vi "Scheduler.Clear-Reset.vi"(7 "All Modules(T)/LocalQ(F)":bool, 8 "error in":errorcluster, 11 "Q In":refnum<queue>) -> (0 "error out":errorcluster, 3 "Q Out":refnum<queue>)   [LabVIEW 2024, in "EQMF.lvlib" / "Scheduler.lvlib"]
uses:
  Scheduler.lvlib
  Queues/Q.Element.ctl
  Queues/Queue Utils.lvlib
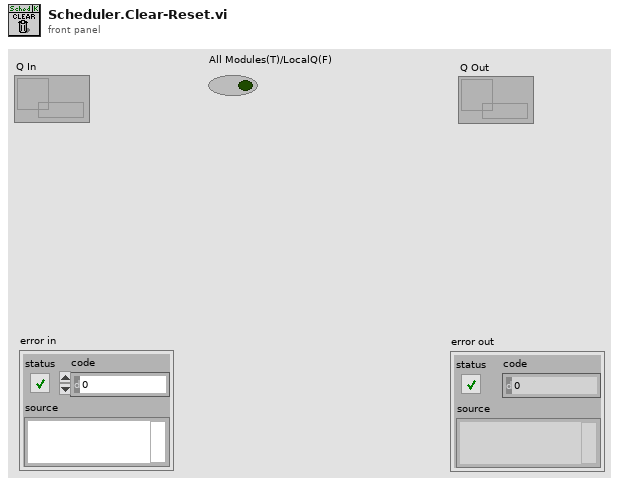
[diagram p1: front panel]
types:
  T1 = typedef "EQMF.lvlib/Queue Utils.lvlib/Q.Element.ctl" = cluster{"Cmd":string, "Sub":string, "Data1":variant, "Data2":variant}
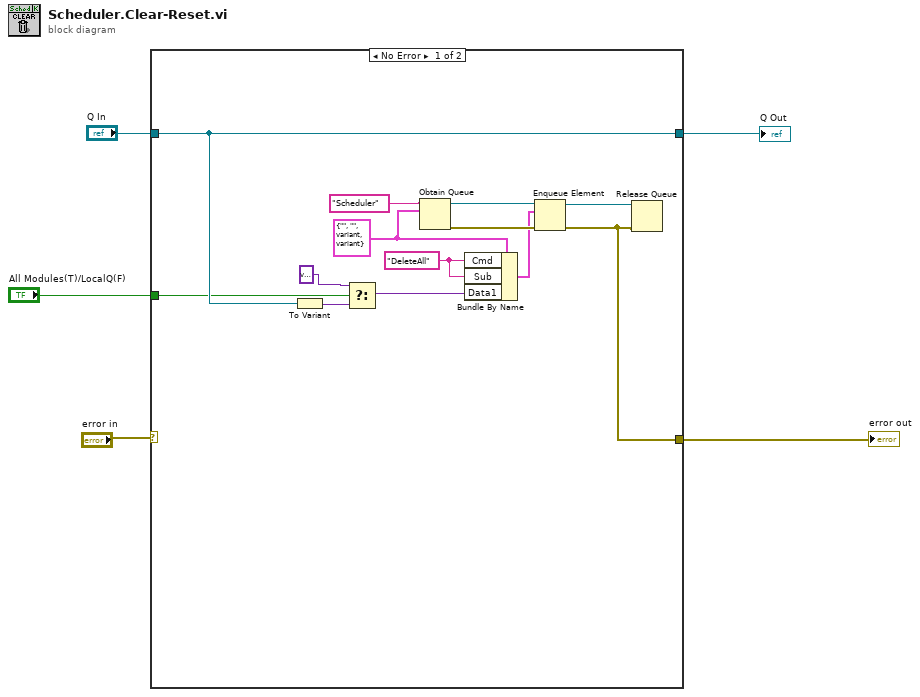
[diagram p0: block diagram]
diagram:
  n1 = case shown="No Error" "error in" {
    selector: "error in" -> [_ w20]
    tunnel: "Q In" -> [w10 w19]
    tunnel: [w15 w20] -> w3
    tunnel: [w10 w19] -> w2
    tunnel: "All Modules(T)/LocalQ(F)" -> [w6 _]
    frame No Error {
      w11 = "DeleteAll" ("Cmd")
      w13 = T1 {"Cmd"="", "Sub"="", "Data1"=variant, "Data2"=variant} ("element")
      n2 = To Variant(anything=w10) -> (Variant=w9:variant)
      n3 = Select(t=variant, s=w6, f=w9) -> (s? t:f=w8:variant)
      n4 = Obtain Queue(name (unnamed)="Scheduler" ("Cmd"), element data type=w13) -> (queue out=w17:refnum<queue>, error out=w16:errorcluster)  [unwired: 3 in, 1 out]
      n5 = Bundle By Name(cluster=w13, "Cmd"=w11, "Sub"=w11, "Data1"=w8) -> (w12:T1)
      n6 = Enqueue Element(queue=w17, element=w12, error in (no error)=w16) -> (queue out=w14:refnum<queue>, error out=w15:errorcluster)  [unwired: 1 in, 1 out]
      n7 = Release Queue(queue=w14, error in (no error)=w15) -> ()  [unwired: 1 in, 3 out]
    }
    frame Error {
    }
  }
  "Q Out" <- w2
  "error out" <- w3
